vi "Add Default Enum.vi"(6 "Hdr Name":T1, 8 "error in (no error)":errorcluster, 9 "Enum Values":u16[](array[numeric]), 11 "Voltage in":refnum<class "Voltage.lvclass">) -> (0 "error out":errorcluster, 3 "Voltage out":refnum<class "Voltage.lvclass">)   [LabVIEW 2012, in "Measurement Channels.lvlib" / "Voltage.lvclass"]
uses:
  Voltage.lvclass
  Common/Controls/HeaderNames.ctl
  Voltage.lvclass/Voltage.ctl
  Class Channel/Read Device.vi
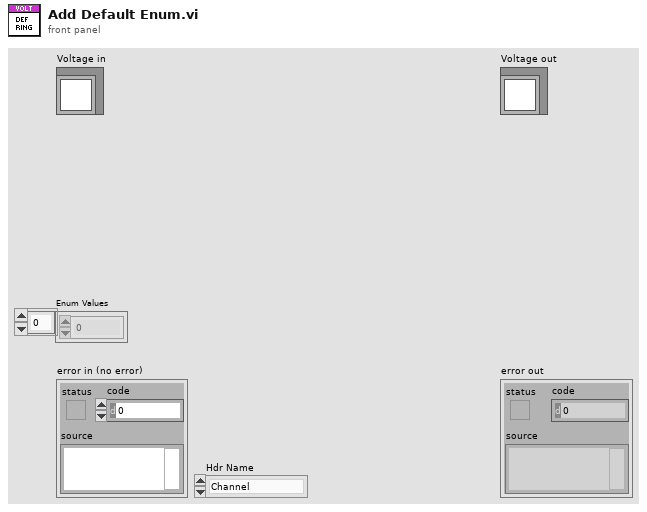
[diagram p1: front panel]
types:
  T1 = typedef "HeaderNames.ctl" = enum16{"Channel", "Device", "Spacer", "Description", "MB", "Range", "Terminal", "Coupling", "Thresh (V)", "Pulse/Rev", "Slope", "Min EU", "Min RPM", "mV/EU", "Iex", "Temp Units", "Type", "CJC Src", "CJC Val", "Ro", "Wire Cfg", "Strain Mode", "Vex", "Bridge Type", "GF", "Gauge Res", "Poisson", "Lead Res", "Init Strain", "GAF", "Scale", "Offset", "Unit (EU)", "dB?", "dB Ref", "Cal Mag", "Cal Units", "Max Temp", "Min Temp", "Max Strain", "Min Strain"}
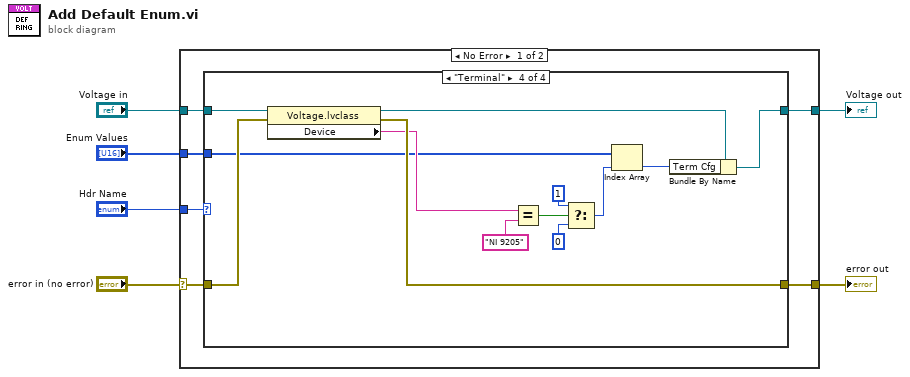
[diagram p0: block diagram]
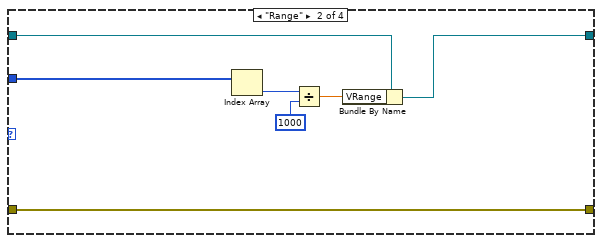
[diagram p3: hidden frame]
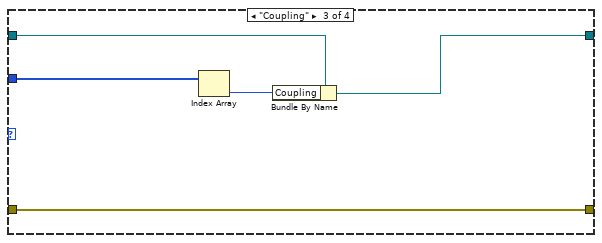
[diagram p4: hidden frame]
diagram:
  n1 = case shown="No Error" "error in (no error)" {
    selector: "error in (no error)" -> [w11 w41]
    tunnel: "Voltage in" -> [w12 w40]
    tunnel: [w10 w40] -> w4
    tunnel: [w9 w41] -> w3
    tunnel: "Hdr Name" -> [w8 _]
    tunnel: "Enum Values" -> [w7 _]
    frame No Error {
      n2 = case shown="\"Terminal\"" w8 {
        tunnel: w12 -> [w14 w21 w25 w39]
        tunnel: w11 -> [w13 w15 w23 w38]
        tunnel: [w14 w20 w24 w36] -> w10
        tunnel: [w13 w15 w23 w35] -> w9
        tunnel: w7 -> [_ w17 w22 w28]
        frame Default {
        }
        frame "Range" {
          n3 = Index Array(array=w17) -> (element=w19:u16)  [unwired: 1 in]
          n4 = Divide(x=w19, y=1000) -> (x/y=w16:dbl)
          n5 = Bundle By Name(cluster=w21, "VRange"=w16) -> (w20:refnum<class "Voltage.lvclass">)
        }
        frame "Coupling" {
          n6 = Index Array(array=w22) -> (element=w26:u16)  [unwired: 1 in]
          n7 = Bundle By Name(cluster=w25, "Coupling"=w26) -> (w24:refnum<class "Voltage.lvclass">)
        }
        frame "Terminal" {
          n8 = property class="Voltage.lvclass"(reference=w39, error in=w38) -> (reference out=w37:refnum<class "Voltage.lvclass">, error out=w35:errorcluster, "Device"=w29:string)
          n9 = Equal?(x=w29, y="NI 9205") -> (x = y?=w32:bool)
          n10 = Select(t=1 ("index"), s=w32, f=0 ("index")) -> (s? t:f=w30:i32)
          n11 = Index Array(array=w28, index=w30) -> (element=w27:u16)
          n12 = Bundle By Name(cluster=w37, "Term Cfg"=w27) -> (w36:refnum<class "Voltage.lvclass">)
        }
      }
    }
    frame Error {
    }
  }
  "error out" <- w3
  "Voltage out" <- w4
